vi "DeltaParameter.vi"(5 "parameter":enum16{"angle", "robot", "vision"}(ring), 7 "mode":enum16{"Read", "Write"}(ring), 8 "error in (no error)":errorcluster, 9 "視覺參數write":T1={"Origin Pixel"={"X"=485.68286, "Y"=264.52893}, "X Axis Pixel"={"X"=485.57736, "Y"=261.4095}, "Axis Reference"=0} {"Axis Reference" items=["Direct", "Indirect"]}, 10 "機構參數write":cluster{"re":dbl, "e":dbl, "rf":dbl, "f":dbl}={"re"=224.0, "e"=38.868, "rf"=145.0, "f"=60.0} {"f" format="%#_13g"; "rf" format="%#_13g"; "e" format="%#_13g"; "re" format="%#_13g"}, 11 "調機參數write":T2={"等比調整到角度正確"={"S1"=1.22, "S2"=1.2, "S3"=1.21, "S4"=5.73, "S5"=0.68}, "補償角度到0度是水平"={"S1"=-50.0, "S2"=-60.0, "S3"=0.0, "S4"=500.0, "S5"=0.0}}) -> (0 "error out":errorcluster, 1 "視覺參數read":T1, 2 "機構參數read":cluster{"re":dbl, "e":dbl, "rf":dbl, "f":dbl}, 3 "調機參數read":T2, 6 "file created?":bool)   [LabVIEW 2019]
uses:
  <vilib>/Utility/config.llb/Read Key (Double).vi
  <vilib>/Utility/config.llb/Write Key (Double).vi
  <vilib>/Utility/config.llb/NI_LVConfig.lvlib
panel:
  out "Numeric":i32
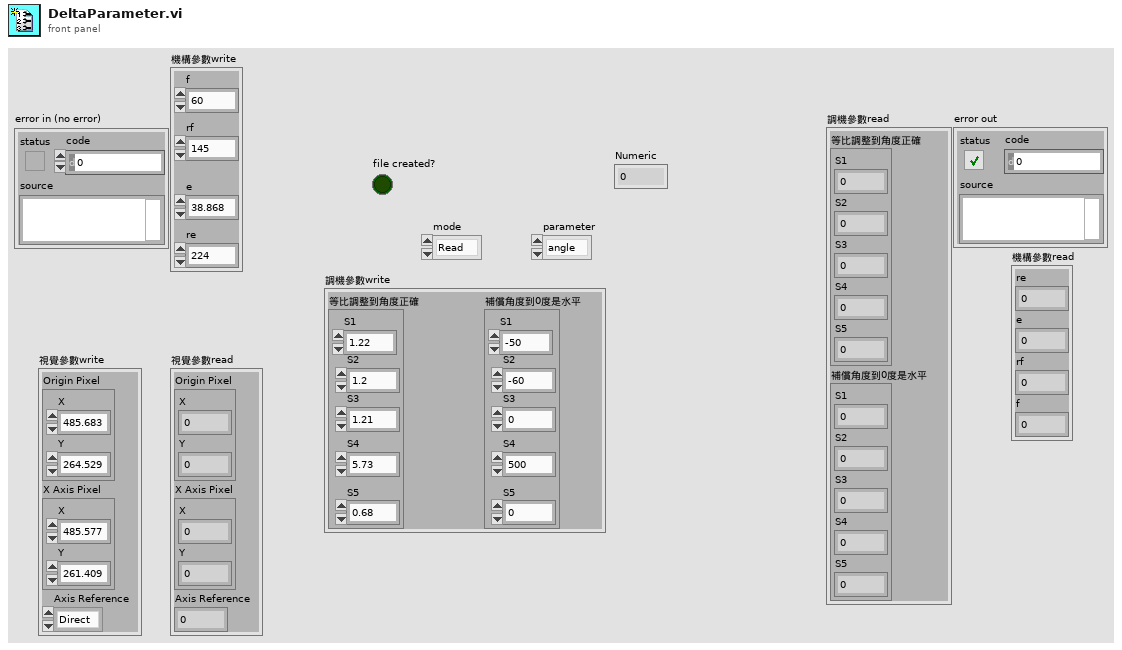
[diagram p1: front panel]
types:
  T1 = cluster{"Origin Pixel":cluster{"X":sgl, "Y":sgl}, "X Axis Pixel":cluster{"X":sgl, "Y":sgl}, "Axis Reference":u32}
  T2 = cluster{"等比調整到角度正確":cluster{"S1":dbl, "S2":dbl, "S3":dbl, "S4":dbl, "S5":dbl}, "補償角度到0度是水平":cluster{"S1":dbl, "S2":dbl, "S3":dbl, "S4":dbl, "S5":dbl}}
  T3 = typedef "NI_LVConfig.lvlib/Config Data RefNum.ctl" = refnum<k1>
  T4 = cluster{"value":dbl, "value":dbl, "value":dbl, "value":dbl, "value":dbl}
  T5 = cluster{"S1":dbl, "S2":dbl, "S3":dbl, "S4":dbl, "S5":dbl}
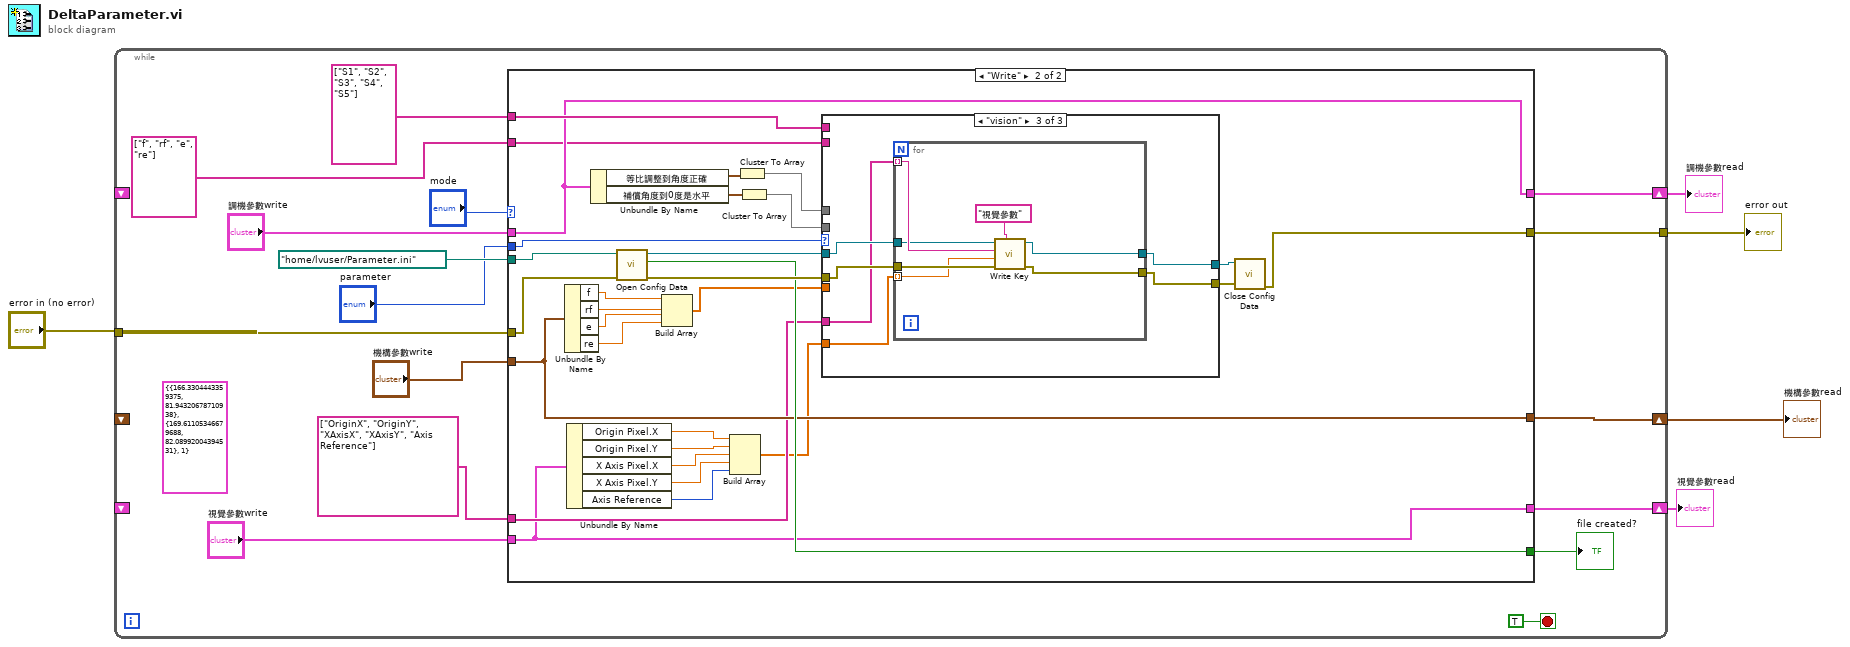
[diagram p0: block diagram]
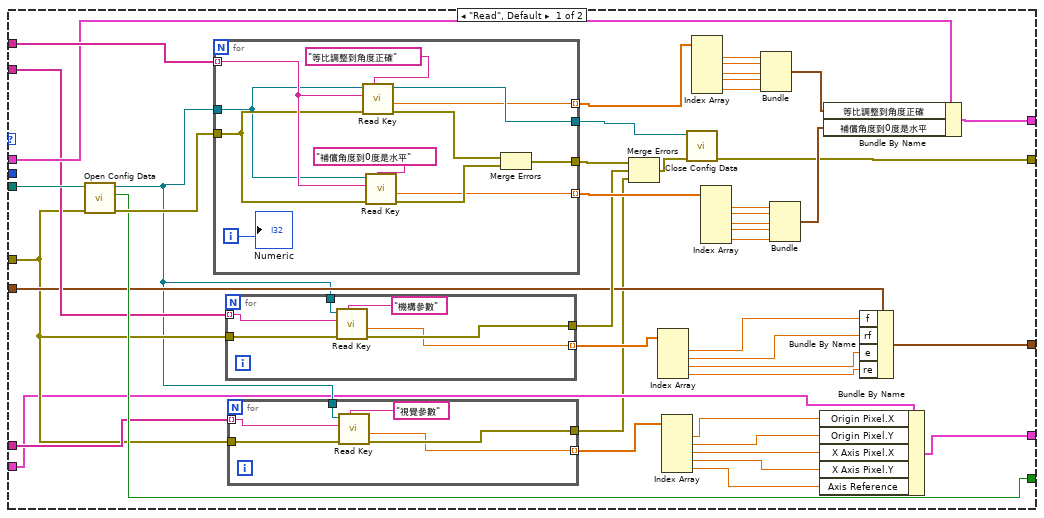
[diagram p2: hidden frame]
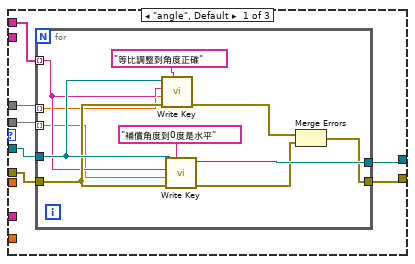
[diagram p3: hidden frame]
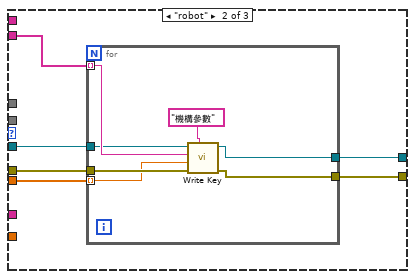
[diagram p4: hidden frame]
diagram:
  n1 = while {
    shift-right: [w16] -> w5
    shift-left: _ -> [_]
    tunnel: [w15] -> w4
    tunnel: "error in (no error)" -> [w14]
    shift-right: [w9] -> w2
    shift-left: _ -> [_]
    shift-right: [w7] -> w1
    shift-left: _ -> [_]
    stop <- TRUE stop-if-true
    (unwired) T1 {"Origin Pixel"={"X"=166.33044, "Y"=81.94321}, "X Axis Pixel"={"X"=169.61105, "Y"=82.08992}, "Axis Reference"=1} ("Calibration Axis Info (Image Calibration 1)")
    n2 = case shown="\"Write\"" "mode" {
      tunnel: path "/home/lvuser/Parameter.ini" ("configuration file path") -> [w65 w112]
      tunnel: string[] ["S1", "S2", "S3", "S4", "S5"] -> [w66 w111]
      tunnel: "調機參數write" -> [w50 w110]
      tunnel: [w49 w110] -> w16
      tunnel: [w46 w108] -> w15
      tunnel: w14 -> [w32 w109]
      tunnel: "parameter" -> [_ w106]
      tunnel: string[] ["f", "rf", "e", "re"] -> [w44 w105]
      tunnel: [w45 w107] -> w11
      tunnel: "機構參數write" -> [w39 w104]
      tunnel: [w34 w104] -> w9
      tunnel: string[] ["OriginX", "OriginY", "XAxisX", "XAxisY", "Axis Reference"] -> [w33 w98]
      tunnel: "視覺參數write" -> [w30 w97]
      tunnel: [w23 w97] -> w7
      frame "Read", Default {
        n3 = call <vilib>:"Open Config Data.vi"("error in (no error)"=w32, "configuration file path"=w65) -> ("error out"=w64:errorcluster, "file created?"=w45:bool, "refnum"=w31:T3)  [unwired: 7 in]
        n4 = for {
          tunnel: w66 -> [w89] mode=indexing
          tunnel: w64 -> [w88]
          tunnel: w31 -> [w87]
          tunnel: [w90] -> w63
          tunnel: [w84] -> w43
          tunnel: [w81] -> w62 mode=indexing
          tunnel: [w80] -> w51 mode=indexing
          i -> [w79]
          n5 = call-poly <vilib>:"Read Key.vi"("section"="等比調整到角度正確", "error in (no error)"=w88, "key"=w89, "refnum"=w87) -> ("error out"=w85:errorcluster, "value"=w81:dbl, "refnum out"=w90:T3)  [unwired: 4 in, 1 out]
          n6 = call-poly <vilib>:"Read Key.vi"("section"="補償角度到0度是水平", "error in (no error)"=w88, "key"=w89, "refnum"=w87) -> ("error out"=w86:errorcluster, "value"=w80:dbl)  [unwired: 4 in, 2 out]
          n7 = Merge Errors(w85, w86) -> (w84:errorcluster)
          "Numeric" <- w79
        }
        n8 = for {
          tunnel: w44 -> [w78] mode=indexing
          tunnel: w31 -> [w77]
          tunnel: w32 -> [w75]
          tunnel: [w74] -> w42
          tunnel: [w73] -> w40 mode=indexing
          n9 = call-poly <vilib>:"Read Key.vi"("section"="機構參數", "error in (no error)"=w75, "key"=w78, "refnum"=w77) -> ("error out"=w74:errorcluster, "value"=w73:dbl)  [unwired: 4 in, 2 out]
        }
        n10 = for {
          tunnel: w33 -> [w72] mode=indexing
          tunnel: w31 -> [w71]
          tunnel: w32 -> [w69]
          tunnel: [w68] -> w22
          tunnel: [w67] -> w29 mode=indexing
          n11 = call-poly <vilib>:"Read Key.vi"("section"="視覺參數", "error in (no error)"=w69, "key"=w72, "refnum"=w71) -> ("error out"=w68:errorcluster, "value"=w67:dbl)  [unwired: 4 in, 2 out]
        }
        n12 = Merge Errors(w43, w42, w22) -> (w41:errorcluster)
        n13 = Index Array(array=w40) -> (element #1=w38:dbl, element #2=w37:dbl, element #3=w36:dbl, element #4=w35:dbl)  [unwired: 4 in]
        n14 = Index Array(array=w29) -> (element #1=w28:dbl, element #2=w27:dbl, element #3=w26:dbl, element #4=w25:dbl, element #5=w24:dbl)  [unwired: 5 in]
        n15 = call <vilib>:"Close Config Data.vi"("error in (no error)"=w41, "refnum"=w63) -> ("error out"=w46:errorcluster)  [unwired: 8 in, 1 out]
        n16 = Index Array(array=w62) -> (element #1=w61:dbl, element #2=w60:dbl, element #3=w59:dbl, element #4=w58:dbl, element #5=w57:dbl)  [unwired: 5 in]
        n17 = Index Array(array=w51) -> (element #1=w52:dbl, element #2=w53:dbl, element #3=w54:dbl, element #4=w55:dbl, element #5=w56:dbl)  [unwired: 5 in]
        n18 = Bundle("value"=w61, "value"=w60, "value"=w59, "value"=w58, "value"=w57) -> (w48:T4)  [unwired: 1 in]
        n19 = Bundle("value"=w52, "value"=w53, "value"=w54, "value"=w55, "value"=w56) -> (w47:T4)  [unwired: 1 in]
        n20 = Bundle By Name(cluster=w30, "Origin Pixel.X"=w28, "Origin Pixel.Y"=w27, "X Axis Pixel.X"=w26, "X Axis Pixel.Y"=w25, "Axis Reference"=w24) -> (w23:T1)
        n21 = Bundle By Name(cluster=w50, "等比調整到角度正確"=w48, "補償角度到0度是水平"=w47) -> (w49:T2)
        n22 = Bundle By Name(cluster=w39, "f"=w38, "rf"=w37, "e"=w36, "re"=w35) -> (w34:cluster{"re":dbl, "e":dbl, "rf":dbl, "f":dbl})
      }
      frame "Write" {
        n23 = Unbundle By Name(w104) -> ("f"=w103:dbl, "rf"=w102:dbl, "e"=w101:dbl, "re"=w100:dbl)
        n24 = Unbundle By Name(w97) -> ("Origin Pixel.X"=w96:sgl, "Origin Pixel.Y"=w95:sgl, "X Axis Pixel.X"=w94:sgl, "X Axis Pixel.Y"=w93:sgl, "Axis Reference"=w92:u32)
        n25 = Unbundle By Name(w110) -> ("等比調整到角度正確"=w116:T5, "補償角度到0度是水平"=w115:T5)
        n26 = call <vilib>:"Open Config Data.vi"("error in (no error)"=w109, "configuration file path"=w112) -> ("error out"=w120:errorcluster, "file created?"=w107:bool, "refnum"=w118:T3)  [unwired: 7 in]
        n27 = Build Array(w103, w102, w101, w100) -> (w99:dbl[])
        n28 = Build Array(w96, w95, w94, w93, w92) -> (w91:sgl[])
        n29 = Cluster To Array(cluster=w116) -> (array=w114:dbl[])
        n30 = Cluster To Array(cluster=w115) -> (array=w113:dbl[])
        n31 = case shown="\"vision\"" w106 {
          tunnel: w120 -> [w123 w142 w157]
          tunnel: [w122 w141 w155] -> w119
          tunnel: w118 -> [w124 w143 w156]
          tunnel: [w121 w140 w154] -> w117
          tunnel: w114 -> [w126 _ _]
          tunnel: w113 -> [w125 _ _]
          tunnel: w111 -> [w127 _ _]
          tunnel: w105 -> [_ w144 _]
          tunnel: w99 -> [_ w139 _]
          tunnel: w98 -> [_ _ w153]
          tunnel: w91 -> [_ _ w152]
          frame "angle", Default {
            n32 = for {
              tunnel: w123 -> [w135]
              tunnel: [w128] -> w122
              tunnel: w124 -> [w136]
              tunnel: [w138] -> w121
              tunnel: w127 -> [w133] mode=indexing
              tunnel: w126 -> [w132] mode=indexing
              tunnel: w125 -> [w131] mode=indexing
              n33 = call-poly <vilib>:"Write Key.vi"("section"="等比調整到角度正確", "error in (no error)"=w135, "value"=w132, "key"=w133, "refnum"=w136) -> ("error out"=w130:errorcluster)  [unwired: 4 in, 2 out]
              n34 = call-poly <vilib>:"Write Key.vi"("section"="補償角度到0度是水平", "error in (no error)"=w135, "value"=w131, "key"=w133, "refnum"=w136) -> ("error out"=w129:errorcluster, "refnum out"=w138:T3)  [unwired: 4 in, 1 out]
              n35 = Merge Errors(w130, w129) -> (w128:errorcluster)
            }
          }
          frame "robot" {
            n36 = for {
              tunnel: w144 -> [w150] mode=indexing
              tunnel: w143 -> [w149]
              tunnel: w142 -> [w148]
              tunnel: [w147] -> w141
              tunnel: [w146] -> w140
              tunnel: w139 -> [w145] mode=indexing
              n37 = call-poly <vilib>:"Write Key.vi"("section"="機構參數", "error in (no error)"=w148, "value"=w145, "key"=w150, "refnum"=w149) -> ("error out"=w147:errorcluster, "refnum out"=w146:T3)  [unwired: 4 in, 1 out]
            }
          }
          frame "vision" {
            n38 = for {
              tunnel: w153 -> [w163] mode=indexing
              tunnel: w156 -> [w162]
              tunnel: w157 -> [w161]
              tunnel: [w160] -> w155
              tunnel: [w159] -> w154
              tunnel: w152 -> [w158] mode=indexing
              n39 = call-poly <vilib>:"Write Key.vi"("section"="視覺參數", "error in (no error)"=w161, "value"=w158, "key"=w163, "refnum"=w162) -> ("error out"=w160:errorcluster, "refnum out"=w159:T3)  [unwired: 4 in, 1 out]
            }
          }
        }
        n40 = call <vilib>:"Close Config Data.vi"("error in (no error)"=w119, "refnum"=w117) -> ("error out"=w108:errorcluster)  [unwired: 8 in, 1 out]
      }
    }
    "file created?" <- w11
  }
  "調機參數read" <- w5
  "error out" <- w4
  "機構參數read" <- w2
  "視覺參數read" <- w1
